vi "Auto Control.vi"   [LabVIEW 2018]
uses:
  <vilib>/Rock Robotics/Network Tables/NT Write String Array.vi
  SubSystems/Drive Train/Drive Train Global.vi
  Robot Global Data.vi
  SubSystems/Hatch Panel Intake/Hatch Panel Intake Global.vi
  SubSystems/Lift/Lift Global.vi
  SubSystems/Cargo Intake/Cargo Intake Global.vi
types:
  T1 = cluster{"X PID":cluster{"proportional gain (Kc)":dbl, "integral time (Ti, min)":dbl, "derivative time (Td, min)":dbl}, "Y PID":cluster{"proportional gain (Kc)":dbl, "integral time (Ti, min)":dbl, "derivative time (Td, min)":dbl}, "Z PID":cluster{"proportional gain (Kc)":dbl, "integral time (Ti, min)":dbl, "derivative time (Td, min)":dbl}}
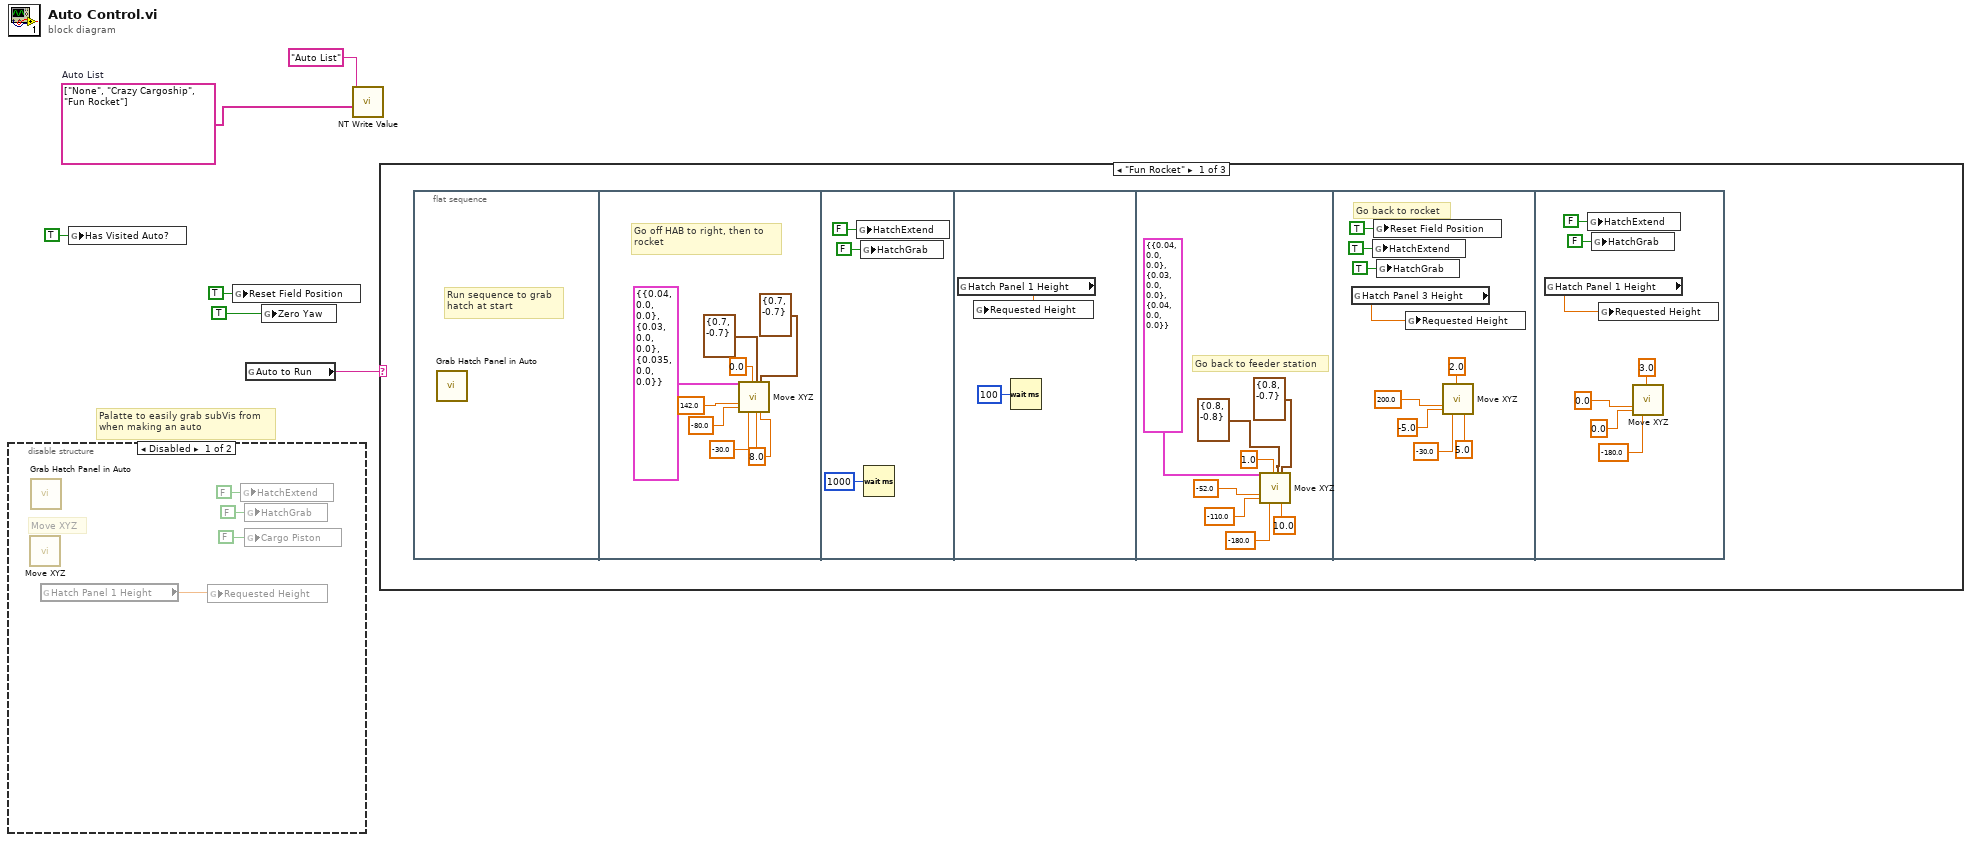
[diagram p0: block diagram]
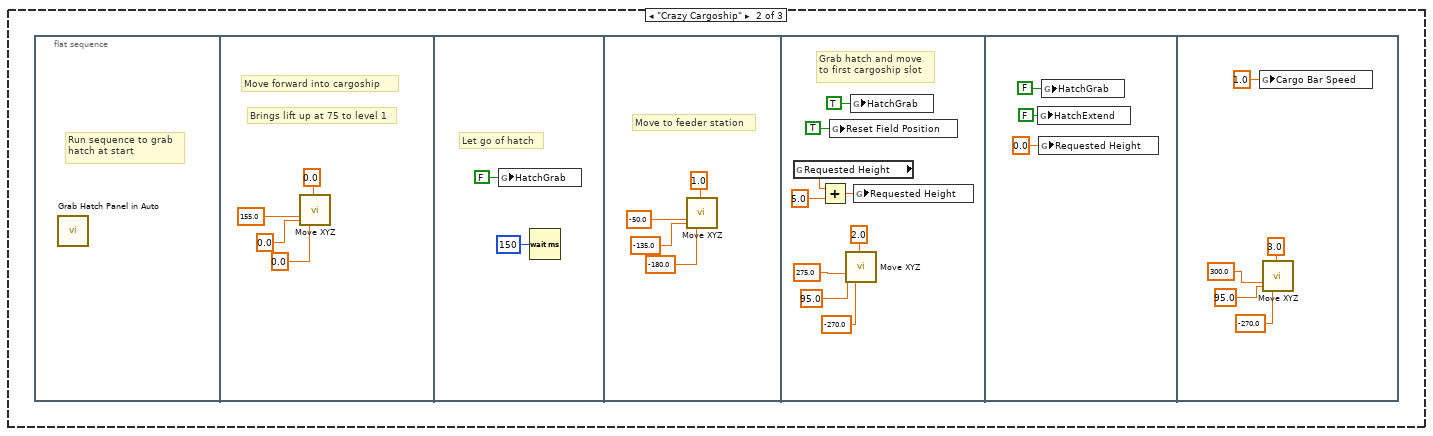
[diagram p3: hidden frame]
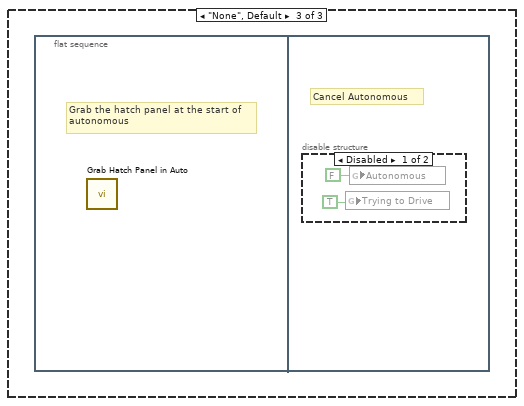
[diagram p4: hidden frame]
diagram:
  w5 = string[] ["None", "Crazy Cargoship", "Fun Rocket"]  # Auto List
  # "Palatte to easily grab subVis from\nwhen making an auto"
  n1 = disable-structure shown="Disabled" {
    frame Disabled {
      # "Move XYZ"
      n2 = call "Move XYZ.vi"() -> ()  [unwired: 28 in]
      n3 = call "Grab Hatch Panel in Auto.vi"() -> ()  [unwired: 12 in]
      n4 = global read "Lift Global.vi" "Hatch Panel 1 Height"() -> (w10:dbl)
      n5 = global write "Lift Global.vi" "Requested Height"(w10) -> ()
      n6 = global write "Hatch Panel Intake Global.vi" "HatchExtend"(FALSE ("HatchExtend")) -> ()
      n7 = global write "Hatch Panel Intake Global.vi" "HatchGrab"(FALSE ("HatchGrab")) -> ()
      n8 = global write "Cargo Intake Global.vi" "Cargo Piston"(FALSE ("Cargo Piston")) -> ()
    }
    frame Enabled {
    }
  }
  n9 = global write "Robot Global Data.vi" "Has Visited Auto?"(TRUE ("Has Visited Auto?")) -> ()
  n10 = global write "Drive Train Global.vi" "Reset Field Position"(TRUE ("Reset Field Position")) -> ()
  n11 = global read "Robot Global Data.vi" "Auto to Run"() -> (w4:string)
  n12 = global write "Drive Train Global.vi" "Zero Yaw"(TRUE ("Reset Field Position")) -> ()
  n13 = call-poly <vilib>:"NT Write Value.vi"("String Array"=w5, "Name"="Auto List") -> ()  [unwired: 9 in, 1 out]
  n14 = case shown="\"Fun Rocket\"" w4 {
    frame "Fun Rocket" {
      n15 = flat-sequence {
        frame #0 {
          # "Run sequence to grab\nhatch at start"
          n16 = call "Grab Hatch Panel in Auto.vi"() -> ()  [unwired: 12 in]
        }
        frame #1 {
          w12 = 8.0 ("X Stop Threshold")
          # "Go off HAB to right, then to\nrocket"
          n17 = call "Move XYZ.vi"("PID Gains In"=T1 {"X PID"={"proportional gain (Kc)"=0.04, "integral time (Ti, min)"=0.0, "derivative time (Td, min)"=0.0}, "Y PID"={"proportional gain (Kc)"=0.03, "integral time (Ti, min)"=0.0, "derivative time (Td, min)"=0.0}, "Z PID"={"proportional gain (Kc)"=0.035, "integral time (Ti, min)"=0.0, "derivative time (Td, min)"=0.0}}, "Y Target"=142.0, "X Target"=-80.0, "Gyro Target"=-30.0, "Movement"=0.0, "X Output Range"=cluster{"output high":dbl, "output low":dbl} {"output high"=0.7, "output low"=-0.7}, "X Stop Threshold"=w12, "Y Output Range"=cluster{"output high":dbl, "output low":dbl} {"output high"=0.7, "output low"=-0.7} ("X Output Range"), "Y Stop Threshold"=w12) -> ()  [unwired: 19 in]
        }
        frame #2 {
          n18 = global write "Hatch Panel Intake Global.vi" "HatchExtend"(FALSE ("HatchExtend")) -> ()
          n19 = global write "Hatch Panel Intake Global.vi" "HatchGrab"(FALSE ("HatchGrab")) -> ()
          n20 = Wait (ms)(milliseconds to wait=u32 1000) -> ()  [unwired: 1 out]
        }
        frame #3 {
          n21 = global read "Lift Global.vi" "Hatch Panel 1 Height"() -> (w23:dbl)
          n22 = global write "Lift Global.vi" "Requested Height"(w23) -> ()
          n23 = Wait (ms)(milliseconds to wait=u32 100) -> ()  [unwired: 1 out]
        }
        frame #4 {
          # "Go back to feeder station"
          n24 = call "Move XYZ.vi"("PID Gains In"=T1 {"X PID"={"proportional gain (Kc)"=0.04, "integral time (Ti, min)"=0.0, "derivative time (Td, min)"=0.0}, "Y PID"={"proportional gain (Kc)"=0.03, "integral time (Ti, min)"=0.0, "derivative time (Td, min)"=0.0}, "Z PID"={"proportional gain (Kc)"=0.04, "integral time (Ti, min)"=0.0, "derivative time (Td, min)"=0.0}}, "Y Target"=-52.0, "X Target"=-110.0, "Gyro Target"=-180.0, "Movement"=1.0, "X Output Range"=cluster{"output high":dbl, "output low":dbl} {"output high"=0.8, "output low"=-0.8}, "Y Output Range"=cluster{"output high":dbl, "output low":dbl} {"output high"=0.8, "output low"=-0.7} ("X Output Range"), "Y Stop Threshold"=10.0) -> ()  [unwired: 20 in]
        }
        frame #5 {
          # "Go back to rocket"
          n25 = global read "Lift Global.vi" "Hatch Panel 3 Height"() -> (w33:dbl)
          n26 = global write "Hatch Panel Intake Global.vi" "HatchExtend"(TRUE ("HatchExtend")) -> ()
          n27 = global write "Drive Train Global.vi" "Reset Field Position"(TRUE ("Reset Field Position")) -> ()
          n28 = global write "Hatch Panel Intake Global.vi" "HatchGrab"(TRUE ("HatchGrab")) -> ()
          n29 = global write "Lift Global.vi" "Requested Height"(w33) -> ()
          n30 = call "Move XYZ.vi"("Y Target"=200.0, "X Target"=-5.0, "Gyro Target"=-30.0, "Movement"=2.0, "Y Stop Threshold"=5.0) -> ()  [unwired: 23 in]
        }
        frame #6 {
          n31 = global read "Lift Global.vi" "Hatch Panel 1 Height"() -> (w45:dbl)
          n32 = global write "Hatch Panel Intake Global.vi" "HatchExtend"(FALSE ("HatchExtend")) -> ()
          n33 = global write "Hatch Panel Intake Global.vi" "HatchGrab"(FALSE ("HatchGrab")) -> ()
          n34 = global write "Lift Global.vi" "Requested Height"(w45) -> ()
          n35 = call "Move XYZ.vi"("Y Target"=0.0, "X Target"=0.0, "Gyro Target"=-180.0, "Movement"=3.0) -> ()  [unwired: 24 in]
        }
      }
    }
    frame "Crazy Cargoship" {
      n36 = flat-sequence {
        frame #0 {
          # "Run sequence to grab\nhatch at start"
          n37 = call "Grab Hatch Panel in Auto.vi"() -> ()  [unwired: 12 in]
        }
        frame #1 {
          # "Brings lift up at 75 to level 1"
          # "Move forward into cargoship"
          n38 = call "Move XYZ.vi"("Y Target"=155.0, "X Target"=0.0, "Gyro Target"=0.0, "Movement"=0.0) -> ()  [unwired: 24 in]
        }
        frame #2 {
          # "Let go of hatch"
          n39 = global write "Hatch Panel Intake Global.vi" "HatchGrab"(FALSE ("HatchGrab")) -> ()
          n40 = Wait (ms)(milliseconds to wait=u32 150) -> ()  [unwired: 1 out]
        }
        frame #3 {
          # "Move to feeder station"
          n41 = call "Move XYZ.vi"("Y Target"=-50.0, "X Target"=-135.0, "Gyro Target"=-180.0, "Movement"=1.0) -> ()  [unwired: 24 in]
        }
        frame #4 {
          # "Grab hatch and move\nto first cargoship slot"
          n42 = global read "Lift Global.vi" "Requested Height"() -> (w62:dbl)
          n43 = Add(x=w62, y=5.0) -> (x+y=w63:dbl)
          n44 = global write "Drive Train Global.vi" "Reset Field Position"(TRUE ("Reset Field Position")) -> ()
          n45 = call "Move XYZ.vi"("Y Target"=275.0, "X Target"=95.0, "Gyro Target"=-270.0, "Movement"=2.0) -> ()  [unwired: 24 in]
          n46 = global write "Hatch Panel Intake Global.vi" "HatchGrab"(TRUE ("HatchGrab")) -> ()
          n47 = global write "Lift Global.vi" "Requested Height"(w63) -> ()
        }
        frame #5 {
          n48 = global write "Hatch Panel Intake Global.vi" "HatchExtend"(FALSE ("HatchGrab")) -> ()
          n49 = global write "Lift Global.vi" "Requested Height"(0.0 ("Requested Height")) -> ()
          n50 = global write "Hatch Panel Intake Global.vi" "HatchGrab"(FALSE ("HatchGrab")) -> ()
        }
        frame #6 {
          n51 = global write "Cargo Intake Global.vi" "Cargo Bar Speed"(1.0 ("Cargo Bar Speed")) -> ()
          n52 = call "Move XYZ.vi"("Y Target"=300.0, "X Target"=95.0, "Gyro Target"=-270.0, "Movement"=3.0) -> ()  [unwired: 24 in]
        }
      }
    }
    frame "None", Default {
      n53 = flat-sequence {
        frame #0 {
          # "Grab the hatch panel at the start of \nautonomous"
          n54 = call "Grab Hatch Panel in Auto.vi"() -> ()  [unwired: 12 in]
        }
        frame #1 {
          # "Cancel Autonomous"
          n55 = disable-structure shown="Disabled" {
            frame Disabled {
              n56 = global write "Robot Global Data.vi" "Trying to Drive"(TRUE ("Autonomous")) -> ()
              n57 = global write "Robot Global Data.vi" "Autonomous"(FALSE ("Autonomous")) -> ()
            }
            frame Enabled {
            }
          }
        }
      }
    }
  }
